vi "Queue Name - Controller.vi"() -> (0 "Queue Name":string="Controller")   [LabVIEW 2016]
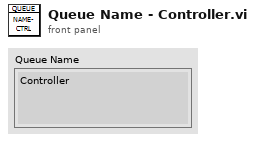
[diagram p1: front panel]
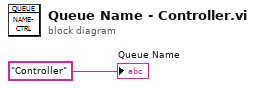
[diagram p0: block diagram]
diagram:
  "Queue Name" <- "Controller"
